vi "Cycle_History_Logging.vi"(8 "error in (no error)":errorcluster, 11 "Diag Cycle String Out":string[][](array[string])) -> (0 "error out":errorcluster)   [LabVIEW 2016]
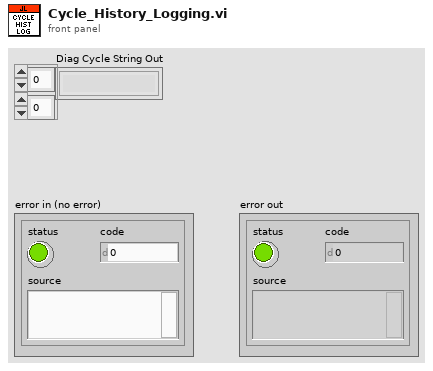
[diagram p1: front panel]
types:
  T1 = enum16{"open", "replace", "create", "open or create", "replace or create", "replace or create with confirmation"}
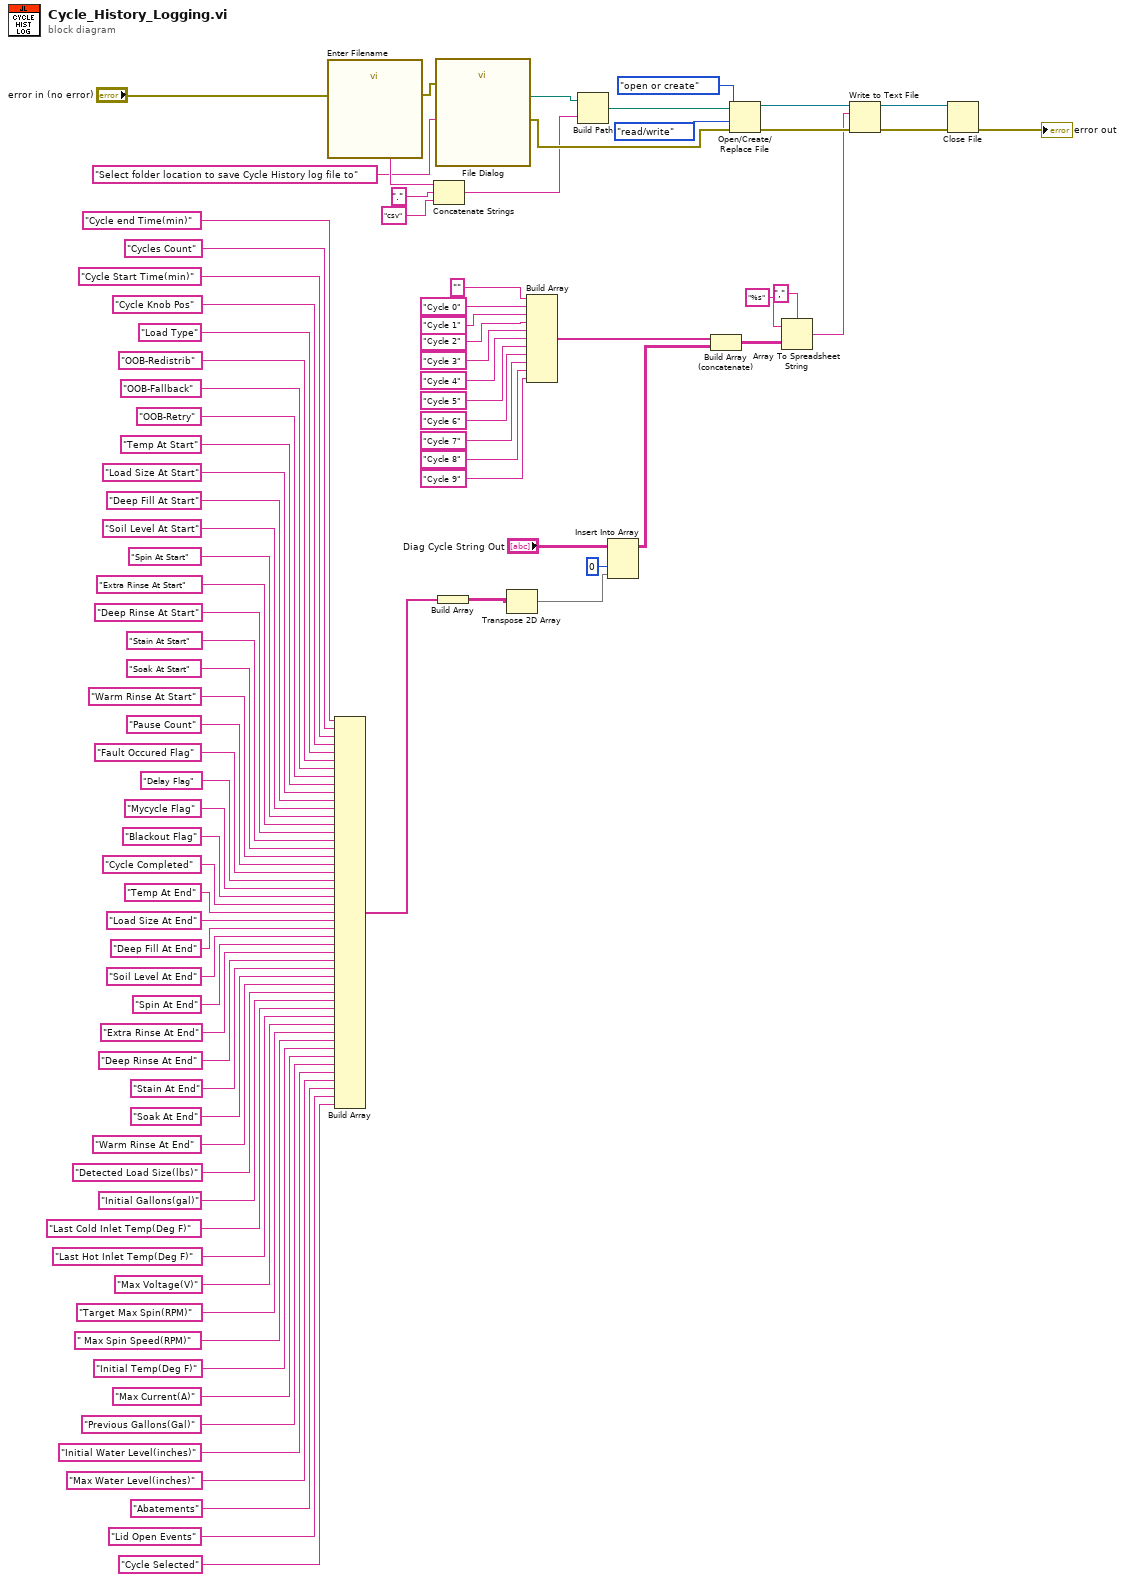
[diagram p0: block diagram]
diagram:
  n1 = call "Enter Filename"("error in (no error)"="error in (no error)") -> ("Filename"=w86:string, "error out"=w81:errorcluster)  [unwired: 16 in, 1 out]
  n2 = Build Array("Cycle end Time(min)" ("delimiter (\\t)"), "Cycles Count" ("delimiter (\\t)"), "Cycle Start Time(min)" ("delimiter (\\t)"), "Cycle Knob Pos" ("delimiter (\\t)"), "Load Type" ("delimiter (\\t)"), "OOB-Redistrib" ("delimiter (\\t)"), "OOB-Fallback" ("delimiter (\\t)"), "OOB-Retry" ("delimiter (\\t)"), "Temp At Start" ("delimiter (\\t)"), "Load Size At Start" ("delimiter (\\t)"), "Deep Fill At Start" ("delimiter (\\t)"), "Soil Level At Start" ("delimiter (\\t)"), "Spin At Start" ("delimiter (\\t)"), "Extra Rinse At Start" ("delimiter (\\t)"), "Deep Rinse At Start" ("delimiter (\\t)"), "Stain At Start" ("delimiter (\\t)"), "Soak At Start" ("delimiter (\\t)"), "Warm Rinse At Start" ("delimiter (\\t)"), "Pause Count" ("delimiter (\\t)"), "Fault Occured Flag" ("delimiter (\\t)"), "Delay Flag" ("delimiter (\\t)"), "Mycycle Flag" ("delimiter (\\t)"), "Blackout Flag" ("delimiter (\\t)"), "Cycle Completed" ("delimiter (\\t)"), "Temp At End" ("delimiter (\\t)"), "Load Size At End" ("delimiter (\\t)"), "Deep Fill At End" ("delimiter (\\t)"), "Soil Level At End" ("delimiter (\\t)"), "Spin At End" ("delimiter (\\t)"), "Extra Rinse At End" ("delimiter (\\t)"), "Deep Rinse At End" ("delimiter (\\t)"), "Stain At End" ("delimiter (\\t)"), "Soak At End" ("delimiter (\\t)"), "Warm Rinse At End" ("delimiter (\\t)"), "Detected Load Size(lbs)" ("delimiter (\\t)"), "Initial Gallons(gal)" ("delimiter (\\t)"), "Last Cold Inlet Temp(Deg F)" ("delimiter (\\t)"), "Last Hot Inlet Temp(Deg F)" ("delimiter (\\t)"), "Max Voltage(V)" ("delimiter (\\t)"), "Target Max Spin(RPM)" ("delimiter (\\t)"), " Max Spin Speed(RPM)" ("delimiter (\\t)"), "Initial Temp(Deg F)" ("delimiter (\\t)"), "Max Current(A)" ("delimiter (\\t)"), "Previous Gallons(Gal)" ("delimiter (\\t)"), "Initial Water Level(inches)" ("delimiter (\\t)"), "Max Water Level(inches)" ("delimiter (\\t)"), "Abatements" ("delimiter (\\t)"), "Lid Open Events" ("delimiter (\\t)"), "Cycle Selected" ("delimiter (\\t)")) -> (w10:string[])
  n3 = Concatenate Strings(w86, "." ("string"), "csv" ("string")) -> (w85:string)
  n4 = call "File Dialog"("prompt"="Select folder location to save Cycle History log file to", "error in"=w81) -> ("selected path"=w18:path, "error out"=w87:errorcluster)  [unwired: 10 in, 2 out]
  n5 = Build Array(w10) -> (w9:string[][])
  n6 = Transpose 2D Array(2D array=w9) -> (transposed array=w3:string[][])
  n7 = Build Array("" ("delimiter (\\t)"), "Cycle 0" ("delimiter (\\t)"), "Cycle 1" ("delimiter (\\t)"), "Cycle 2" ("delimiter (\\t)"), "Cycle 3" ("delimiter (\\t)"), "Cycle 4" ("delimiter (\\t)"), "Cycle 5" ("delimiter (\\t)"), "Cycle 6" ("delimiter (\\t)"), "Cycle 7" ("delimiter (\\t)"), "Cycle 8" ("delimiter (\\t)"), "Cycle 9" ("delimiter (\\t)")) -> (w13:string[])
  n8 = Build Path(base path=w18, name or relative path=w85) -> (appended path=w67:path)
  n9 = Insert Into Array(array="Diag Cycle String Out", index (col)=0 ("disabled index (col)"), new element=w3) -> (w4:string[][])  [unwired: 1 in]
  n10 = Build Array (concatenate)(w13, w4) -> (w12:string[][])
  n11 = Open/Create/Replace File(file path (use dialog)=w67, error in=w87, operation (0:open)=T1."open or create", access (0:read/write)=enum16{"read/write", "read-only", "write-only"}."read/write") -> (refnum out=w17:refnum<file>, error out=w16:errorcluster)  [unwired: 2 in, 1 out]
  n12 = Array To Spreadsheet String(delimiter (Tab)=",", array=w12, 3:"%s" ("format string")) -> (spreadsheet string=w11:string)
  n13 = Write to Text File(file (use dialog)=w17, text=w11, error in=w16) -> (refnum out=w8:refnum<file>, error out=w7:errorcluster)  [unwired: 1 in, 1 out]
  n14 = Close File(refnum=w8, error in=w7) -> (error out=→"error out":errorcluster)  [unwired: 1 out]
